vi "[FGV] Output List.vi"(7 "Action":T2(ring), 8 "error in (no error)":errorcluster, 9 "Criteria":string[](array[string]), 10 "Indexes In":u16[](array[numeric])) -> (0 "error out":errorcluster, 2 "Output":T1)   [LabVIEW 2019]
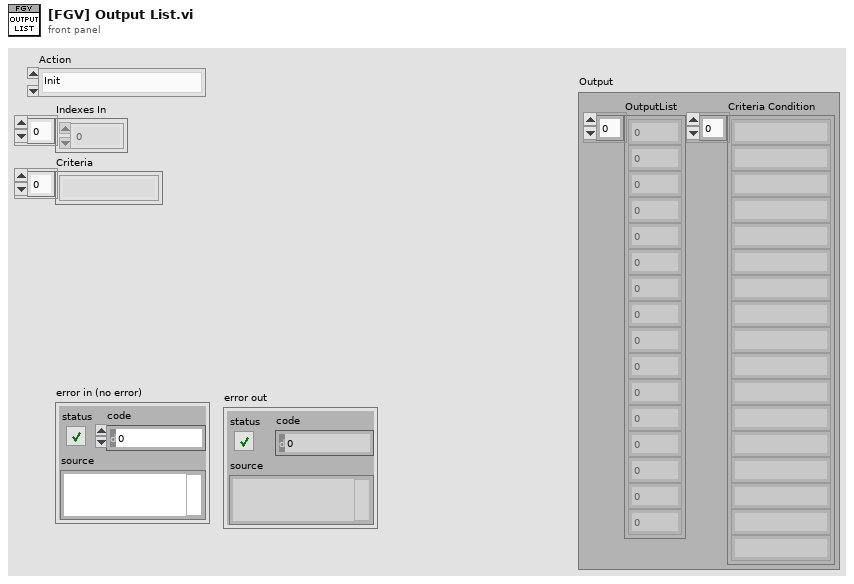
[diagram p1: front panel]
types:
  T1 = cluster{"OutputList":u16[], "Criteria Condition":string[]}
  T2 = enum16{"Init", "Add", "Remove", "Read All", "Remove All", "WriteCriteria"}
  T3 = cluster{"Index":u16[], "Criteria Condition":string[]}
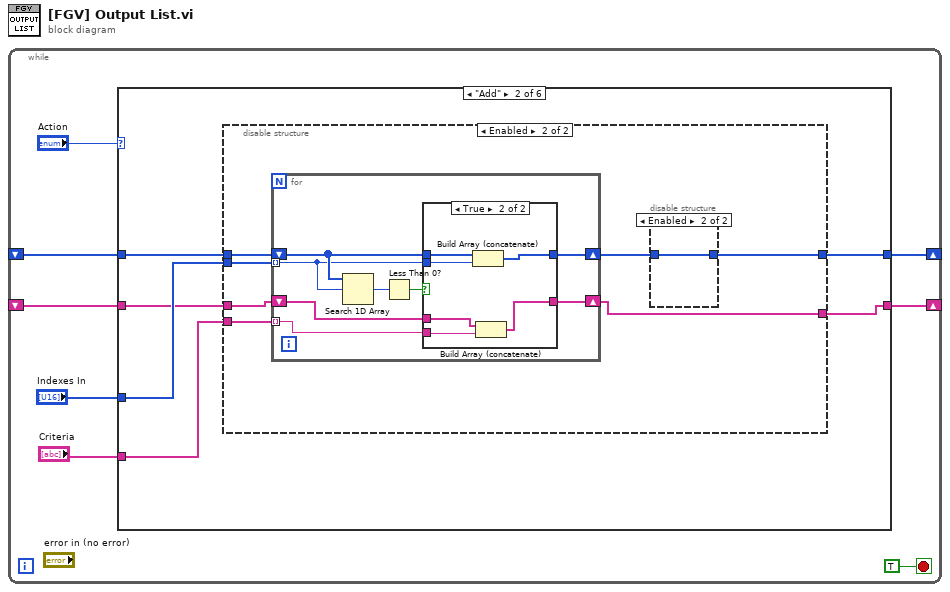
[diagram p0: block diagram]
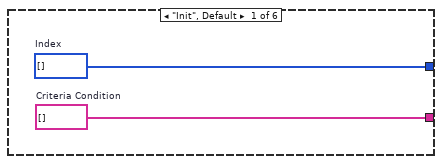
[diagram p2: hidden frame]
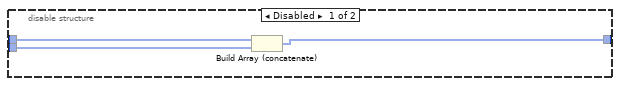
[diagram p3: hidden frame]
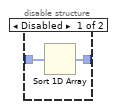
[diagram p4: hidden frame]
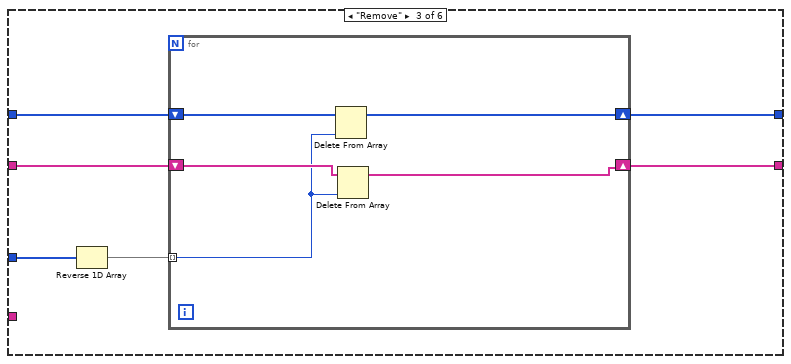
[diagram p6: hidden frame]
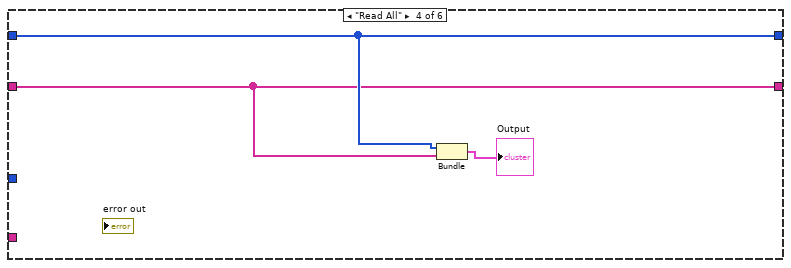
[diagram p7: hidden frame]
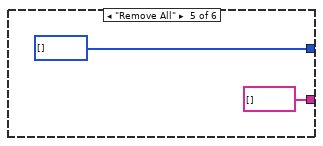
[diagram p8: hidden frame]
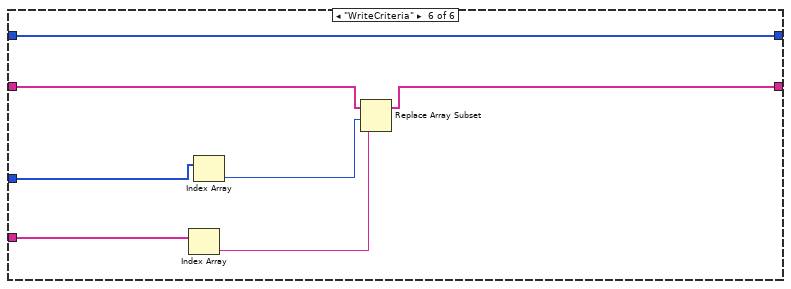
[diagram p9: hidden frame]
diagram:
  n1 = while {
    shift-right: [w6] -> _
    shift-left: _ -> [w5]
    shift-right: [w3] -> _
    shift-left: _ -> [w2]
    stop <- TRUE stop-if-true
    n2 = case shown="\"Add\"" "Action" {
      tunnel: [w10 w15 w48 w59 u16[] [] w68] -> w6
      tunnel: w5 -> [_ w16 w49 w59 _ w68]
      tunnel: "Indexes In" -> [_ w14 w51 _ _ w65]
      tunnel: [w9 w12 w46 w58 string[] [] ("Criteria Condition") w66] -> w3
      tunnel: w2 -> [_ w13 w47 w58 _ w67]
      tunnel: "Criteria" -> [_ w11 _ _ _ w63]
      frame "Init", Default {
        w9 = string[] []  # Criteria Condition
        w10 = u16[] []  # Index
      }
      frame "Add" {
        n3 = disable-structure shown="Enabled" {
          disable-tunnel: w16 -> [w19 w25]
          disable-tunnel: [w18 w23] -> w15
          disable-tunnel: w14 -> [w17 w26]
          disable-tunnel: w13 -> [_ w22]
          disable-tunnel: [_ w21] -> w12
          disable-tunnel: w11 -> [_ w20]
          frame Disabled {
            n4 = Build Array (concatenate)(w19, w17) -> (w18:u16[])
          }
          frame Enabled {
            n5 = for {
              tunnel: w26 -> [w33] mode=indexing
              shift-right: [w34] -> w24
              shift-left: w25 -> [w35]
              shift-right: [w31] -> w21
              shift-left: w22 -> [w32]
              tunnel: w20 -> [w30] mode=indexing
              n6 = Search 1D Array(1D array=w35, element=w33) -> (index of element=w37:i32)  [unwired: 1 in]
              n7 = Less Than 0?(x=w37) -> (x < 0?=w36:bool)
              n8 = case shown="True" w36 {
                tunnel: w35 -> [w39 w45]
                tunnel: [w39 w44] -> w34
                tunnel: w33 -> [_ w43]
                tunnel: w32 -> [w38 w42]
                tunnel: [w38 w41] -> w31
                tunnel: w30 -> [_ w40]
                frame False {
                }
                frame True {
                  n9 = Build Array (concatenate)(w45, w43) -> (w44:u16[])
                  n10 = Build Array (concatenate)(w42, w40) -> (w41:string[])
                }
              }
            }
            n11 = disable-structure shown="Enabled" {
              disable-tunnel: w24 -> [w28 w29]
              disable-tunnel: [w27 w29] -> w23
              frame Disabled {
                n12 = Sort 1D Array(array=w28) -> (sorted array=w27:u16[])
              }
              frame Enabled {
              }
            }
          }
        }
      }
      frame "Remove" {
        n13 = Reverse 1D Array(array=w51) -> (reversed array=w50:u16[])
        n14 = for {
          tunnel: w50 -> [w53] mode=indexing
          shift-right: [w55] -> w48
          shift-left: w49 -> [w56]
          shift-right: [w52] -> w46
          shift-left: w47 -> [w54]
          n15 = Delete From Array(array=w56, index=w53) -> (array with subset deleted=w55:u16[])  [unwired: 1 in, 1 out]
          n16 = Delete From Array(array=w54, index=w53) -> (array with subset deleted=w52:string[])  [unwired: 1 in, 1 out]
        }
      }
      frame "Read All" {
        n17 = Bundle("Index"=w59, "Criteria Condition"=w58) -> (→"Output":T3)  [unwired: 1 in]
      }
      frame "Remove All" {
      }
      frame "WriteCriteria" {
        n18 = Index Array(array=w63) -> (element=w62:string)  [unwired: 1 in]
        n19 = Index Array(array=w65) -> (element=w64:u16)  [unwired: 1 in]
        n20 = Replace Array Subset(array=w67, new element=w62, index=w64) -> (w66:string[])
      }
    }
  }
